vi "Create TCP Connection.vi"(5 "TCPConnection in":refnum<class "TCPConnection.lvclass">, 8 "error in (no error)":errorcluster, 11 "connection ID":refnum<k5>) -> (0 "error out":errorcluster, 3 "TCPConnection out":refnum<class "TCPConnection.lvclass">)   [LabVIEW 2013, in "MQTT Server.lvlib" / "TCPConnection.lvclass"]
uses:
  TCPConnection.lvclass
  TCPConnection.lvclass/TCPConnection.ctl
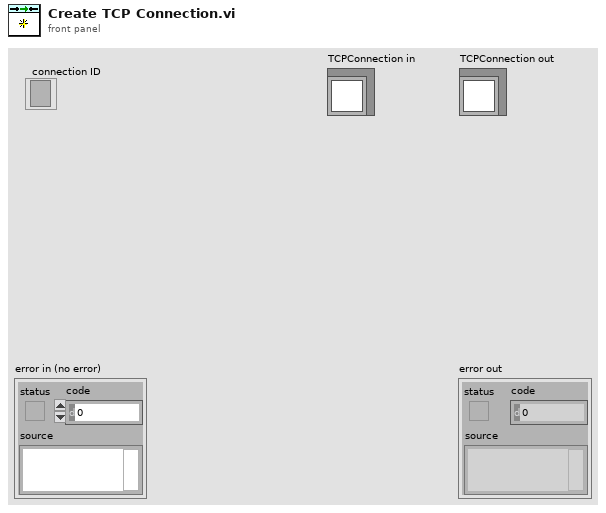
[diagram p1: front panel]
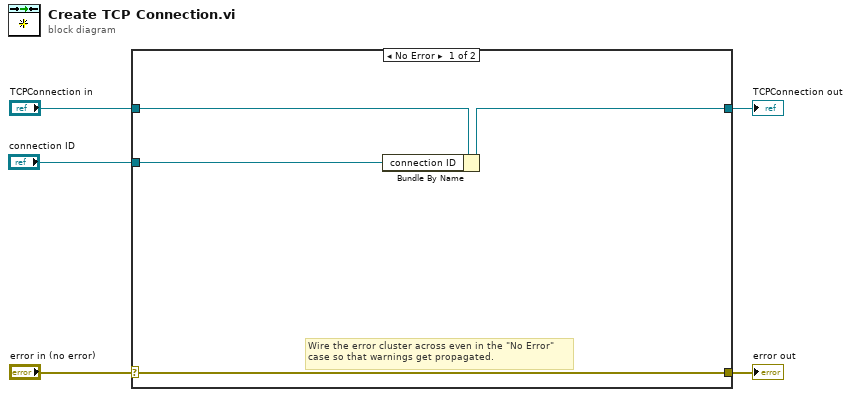
[diagram p0: block diagram]
diagram:
  n1 = case shown="No Error" "error in (no error)" {
    selector: "error in (no error)" -> [w8 w11]
    tunnel: [w8 w11] -> w4
    tunnel: [w7 w10] -> w2
    tunnel: "TCPConnection in" -> [w9 w10]
    tunnel: "connection ID" -> [w6 _]
    frame No Error {
      # "Wire the error cluster across even in the \"No Error\"\ncase so that warnings get propagated."
      n2 = Bundle By Name(cluster=w9, "connection ID"=w6) -> (w7:refnum<class "TCPConnection.lvclass">)
    }
    frame Error {
    }
  }
  "error out" <- w4
  "TCPConnection out" <- w2
